vi "Move.vi"(8 "error in (no error)":errorcluster, 11 "AISAS Mech in":refnum<class "AISAS Mech.lvclass">) -> (0 "error out":errorcluster, 3 "AISAS Mech out":refnum<class "AISAS Mech.lvclass">, 5 "status log":string)   [LabVIEW 2014, in "AISAS Mech.lvclass"]
uses:
  AISAS Mech.lvclass
  AISAS Mech.lvclass/AISAS Mech.ctl
  motor/Motor status.ctl
  motor/AISAS motor.lvclass
panel:
  out "M name":string
  in  "Abort":bool
  out "Elapsed Time (s)":dbl
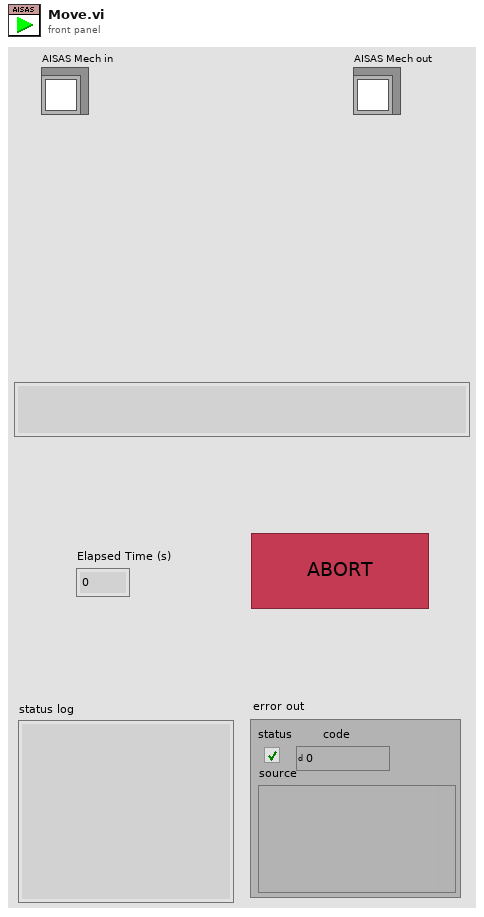
[diagram p1: front panel]
types:
  T1 = typedef "AISAS motor.lvclass/Motor status.ctl" = enum16{"Error", "Ready", "Bussy"}
  T2 = typedef "motor.ctl" = enum32{"Rotation", "Diffuser ", "Focus"}
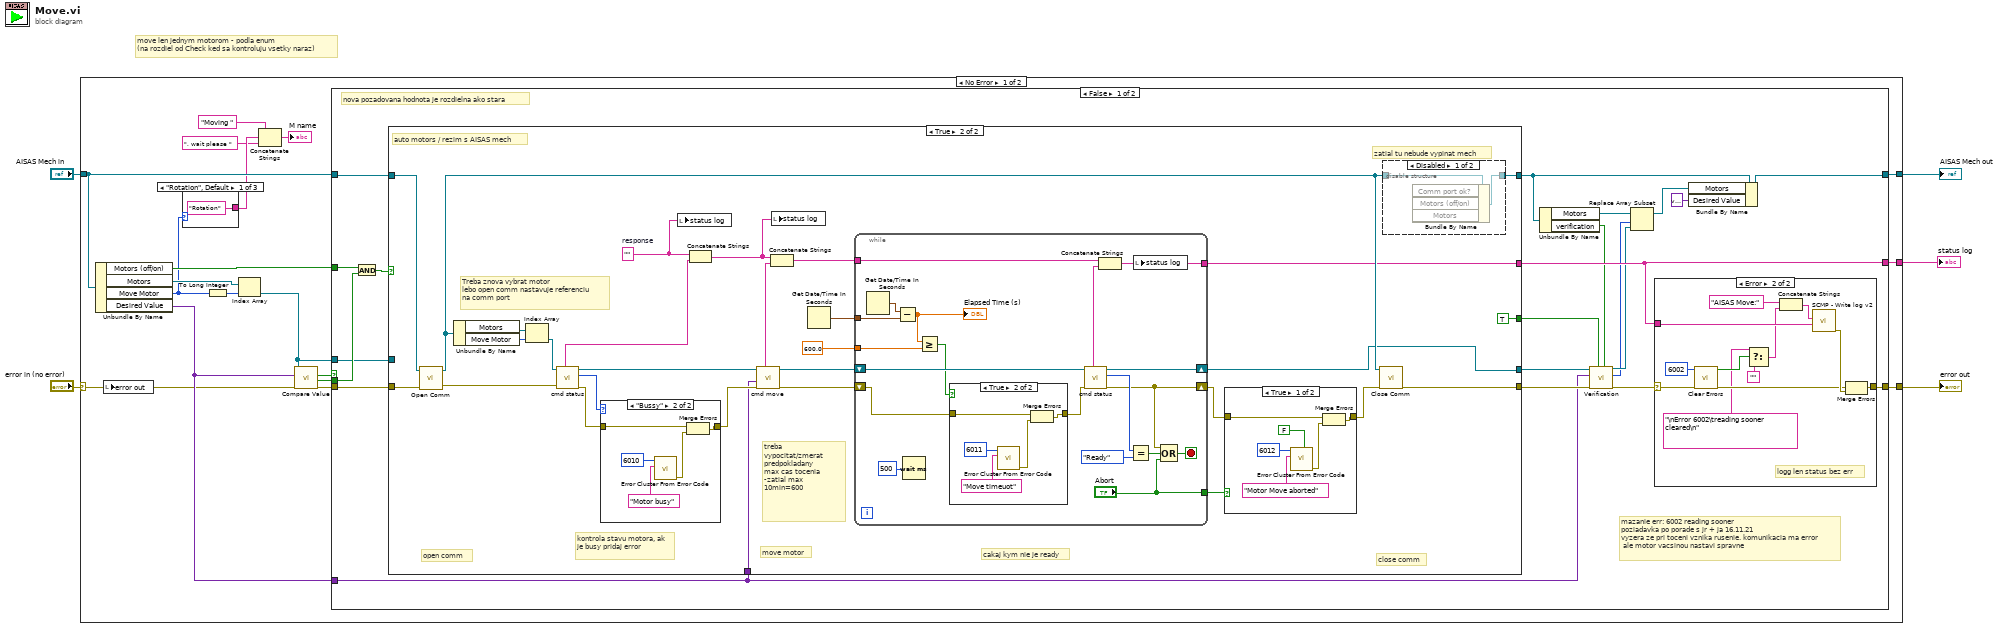
[diagram p0: block diagram]
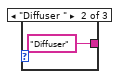
[diagram p2: hidden frame]
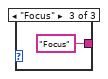
[diagram p3: hidden frame]
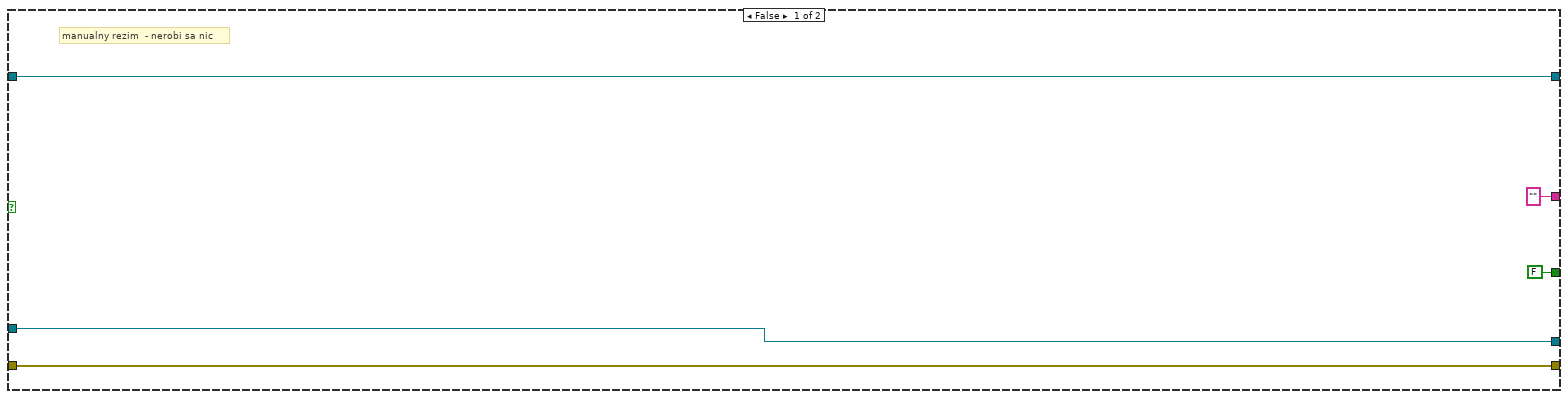
[diagram p5: hidden frame]
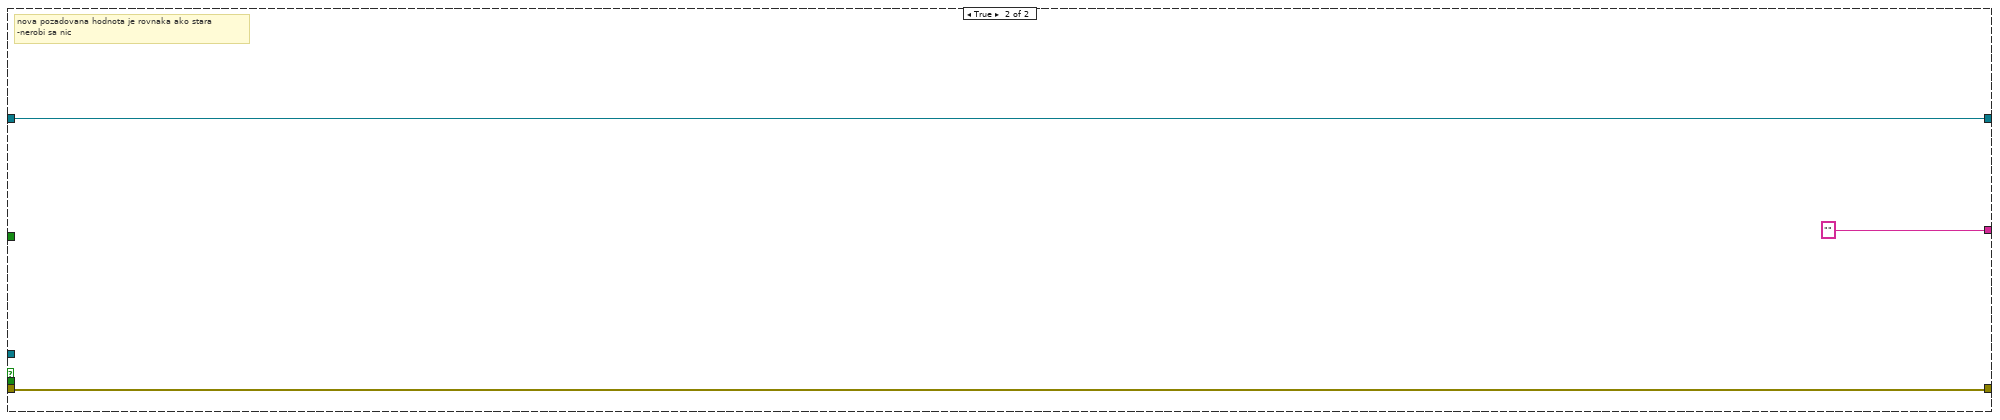
[diagram p10: hidden frame]
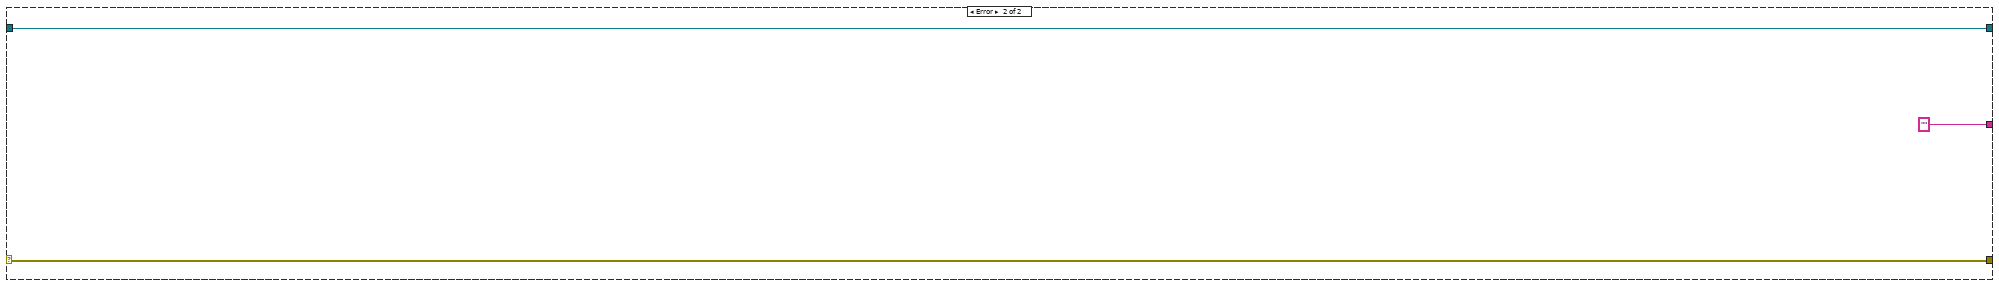
[diagram p11: hidden frame]
diagram:
  # "move len jednym motorom - podla enum \n(na rozdiel od Check ked sa kontroluju vsetky naraz)"
  n1 = case shown="No Error" "error in (no error)" {
    selector: "error in (no error)" -> [w12 w141]
    tunnel: [w23 w141] -> w5
    tunnel: "AISAS Mech in" -> [w21 w140]
    tunnel: [w22 w140] -> w2
    tunnel: [w15 ""] -> w1
    frame No Error {
      n2 = Unbundle By Name(w21) -> ("Motors (off/on)"=w18:bool, "Motors"=w16:refnum<class "AISAS motor.lvclass">[], "Move Motor"=w10:T2, "Desired Value"=w13:variant)
      n3 = local write "error out"(w12) -> ()
      n4 = case shown="\"Rotation\", Default" w10 {
        tunnel: ["Rotation" ("M name") "Diffuser" ("M name") "Focus" ("M name")] -> w8
        frame "Rotation", Default {
        }
        frame "Diffuser " {
        }
        frame "Focus" {
        }
      }
      n5 = To Long Integer(number=w10) -> (32bit integer=w11:i32)
      n6 = Index Array(array=w16, index=w11) -> (element=w14:refnum<class "AISAS motor.lvclass">)
      n7 = Concatenate Strings("Moving " ("M name"), w8, ", wait please " ("M name")) -> (→"M name":string)
      n8 = call "Compare Value.vi"("error in (no error)"=w12, "new Value"=w13, "AISAS motor in"=w14) -> ("error out"=w17:errorcluster, "Motor Ok?"=w19:bool, "same value?"=w20:bool)  [unwired: 3 in, 3 out]
      n9 = case shown="False" w20 {
        tunnel: [w31 w137] -> w23
        tunnel: [w40 w138] -> w22
        tunnel: w21 -> [w47 w138]
        tunnel: w19 -> [w39 _]
        tunnel: w18 -> [w46 _]
        tunnel: w17 -> [w44 w137]
        tunnel: [w30 ""] -> w15
        tunnel: w14 -> [w38 _]
        tunnel: w13 -> [w33 _]
        frame False {
          # "mazanie err: 6002\treading sooner\npoziadavka po porade s jr + ja 16.11.21\nvyzera ze pri toceni vznika rusenie. komunikacia ma error\n ale motor vacsinou nastavi spravne"
          # "nova pozadovana hodnota je rozdielna ako stara"
          n10 = And(x=w46, y=w39) -> (x .and. y?=w45:bool)
          n11 = case shown="True" w45 {
            tunnel: [w64 w74] -> w37
            tunnel: w47 -> [w65 w83]
            tunnel: [w65 w94] -> w41
            tunnel: w44 -> [w64 w85]
            tunnel: [w62 w78] -> w36
            tunnel: ["" w67] -> w30
            tunnel: w38 -> [w62 _]
            tunnel: [FALSE ("Motor (man/auto)") TRUE ("Motor (man/auto)")] -> w35
            tunnel: w33 -> [_ w75]
            frame False {
              # "manualny rezim  - nerobi sa nic"
            }
            frame True {
              w70 = ""  # response
              # "Treba znova vybrat motor\nlebo open comm nastavuje referenciu\nna comm port"
              # "close comm"
              # "cakaj kym nie je ready"
              # "move motor"
              # "kontrola stavu motora, ak je busy pridaj error"
              # "zatial tu nebude vypinat mech"
              # "treba \nvypocitat/zmerat \npredpokladany\nmax cas tocenia\n-zatial max 10min=600"
              # "auto motors / rezim s AISAS mech"
              # "open comm"
              n12 = call "Open Comm.vi"("error in (no error)"=w85, "AISAS Mech in"=w83) -> ("error out"=w84:errorcluster, "AISAS Mech out"=w80:refnum<class "AISAS Mech.lvclass">)  [unwired: 7 in, 1 out]
              n13 = Unbundle By Name(w80) -> ("Motors"=w82:refnum<class "AISAS motor.lvclass">[], "Move Motor"=w76:T2)
              n14 = Index Array(array=w82, index=w76) -> (element=w81:refnum<class "AISAS motor.lvclass">)
              n15 = call "cmd status.vi"("error in (no error)"=w84, "motor in"=w81) -> ("error out"=w86:errorcluster, "Motor status"=w79:T1, "motor out"=w93:refnum<class "AISAS motor.lvclass">, "status log"=w89:string)  [unwired: 5 in, 1 out]
              n16 = case shown="\"Bussy\"" w79 {
                tunnel: w86 -> [w130 w133]
                tunnel: [w130 w131] -> w92
                frame "Error", Default {
                }
                frame "Bussy" {
                  n17 = call <vilib>:"Error Cluster From Error Code.vi"("error message (\"\")"="Motor busy" ("error message (\"\")"), "error code (0)"=6010) -> ("error out"=w132:errorcluster)  [unwired: 7 in]
                  n18 = Merge Errors(w133, w132) -> (w131:errorcluster)
                }
              }
              n19 = local write "status log"(w70) -> ()
              n20 = Concatenate Strings(w70, w89) -> (w69:string)
              n21 = call "cmd move.vi"("error in (no error)"=w92, "new Value"=w75, "motor in"=w93) -> ("error out"=w91:errorcluster, "motor out"=w90:refnum<class "AISAS motor.lvclass">, "Log response"=w88:string)  [unwired: 4 in, 2 out]
              n22 = Concatenate Strings(w69, w88) -> (w68:string)
              n23 = local write "status log"(w69) -> ()
              n24 = Get Date/Time In Seconds() -> (seconds since 1Jan1904=w66:timestamp)
              n25 = while {
                shift-right: [w117] -> w72
                shift-left: w91 -> [w106]
                shift-right: [w120] -> w78
                shift-left: w90 -> [w121]
                tunnel: 600.0 ("Time Target (s)") -> [w109]
                tunnel: ["Abort"] -> w73
                tunnel: w68 -> [w114]
                tunnel: [w112] -> w67
                tunnel: w66 -> [w111]
                stop <- w116 stop-if-true
                n26 = Get Date/Time In Seconds() -> (seconds since 1Jan1904=w110:timestamp)
                n27 = Subtract(x=w110, y=w111) -> (x-y=w108:dbl)
                "Elapsed Time (s)" <- w108
                n28 = Wait (ms)(milliseconds to wait=u32 500) -> ()  [unwired: 1 out]
                n29 = Greater Or Equal?(x=w108, y=w109) -> (x >= y?=w107:bool)
                n30 = case shown="True" w107 {
                  tunnel: [w124 w127] -> w122
                  tunnel: w106 -> [w124 w125]
                  frame False {
                  }
                  frame True {
                    n31 = call <vilib>:"Error Cluster From Error Code.vi"("error message (\"\")"="Move timeuot" ("error message (\"\")"), "error code (0)"=6011) -> ("error out"=w126:errorcluster)  [unwired: 7 in]
                    n32 = Merge Errors(w125, w126) -> (w127:errorcluster)
                  }
                }
                n33 = call "cmd status.vi"("error in (no error)"=w122, "motor in"=w121) -> ("error out"=w117:errorcluster, "Motor status"=w119:T1, "motor out"=w120:refnum<class "AISAS motor.lvclass">, "status log"=w113:string)  [unwired: 5 in, 1 out]
                n34 = Concatenate Strings(w114, w113) -> (w112:string)
                n35 = Equal?(x=w119, y=Motor_status."Ready") -> (x = y?=w115:bool)
                n36 = local write "status log"(w112) -> ()
                n37 = Compound Arithmetic op=OR(w117, w115, "Abort") -> (w116:bool)
              }
              n38 = case shown="True" w73 {
                tunnel: w72 -> [w98 w101]
                tunnel: [w96 w101] -> w71
                frame True {
                  n39 = call <vilib>:"Error Cluster From Error Code.vi"("is warning? (False)"=FALSE, "error message (\"\")"="Motor Move aborted" ("error message (\"\")"), "error code (0)"=6012) -> ("error out"=w97:errorcluster)  [unwired: 6 in]
                  n40 = Merge Errors(w98, w97) -> (w96:errorcluster)
                }
                frame False {
                }
              }
              n41 = call "Close Comm.vi"("error in (no error)"=w71, "AISAS Mech"=w80) -> ("error out"=w74:errorcluster)  [unwired: 9 in]
              n42 = disable-structure shown="Disabled" {
                disable-tunnel: w80 -> [w103 w104]
                disable-tunnel: [w102 w104] -> w94
                frame Disabled {
                  n43 = Bundle By Name(cluster=w103) -> (w102:refnum<class "AISAS Mech.lvclass">)  [unwired: 3 in]
                }
                frame Enabled {
                }
              }
            }
          }
          n44 = Unbundle By Name(w41) -> ("Motors"=w43:refnum<class "AISAS motor.lvclass">[], "verification"=w27:bool)
          n45 = call "Verification.vi"("verification"=w27, "Motor\n(man/auto)"=w35, "error in (no error)"=w37, "Value in"=w33, "AISAS motor in"=w36) -> ("error out"=w32:errorcluster, "Motor"=w28:T2, "AISAS motor out"=w29:refnum<class "AISAS motor.lvclass">)  [unwired: 4 in]
          n46 = Replace Array Subset(array=w43, new element=w29, index=w28) -> (w42:refnum<class "AISAS motor.lvclass">[])
          n47 = case shown="Error" w32 {
            selector: w32 -> [w48 w56]
            tunnel: [w48 w58] -> w31
            tunnel: w30 -> [_ w60]
            frame No Error {
            }
            frame Error {
              # "logg len status bez err"
              n48 = call <vilib>:"Clear Errors.vi"("error in (no error)"=w56, "specific error code to clear (0: all)"=6002) -> ("error out"=w55:errorcluster, "specific error cleared?"=w54:bool)  [unwired: 4 in]
              n49 = Select(t="\nError 6002\treading sooner cleared\n" ("data"), s=w54, f="") -> (s? t:f=w51:string)
              n50 = Concatenate Strings("AISAS Move:" ("data"), w51) -> (w52:string)
              n51 = call "SCMP - Write log v2.vi"("data to end"=w60, "data"=w52) -> ("error out"=w59:errorcluster)  [unwired: 7 in, 2 out]
              n52 = Merge Errors(w55, w59) -> (w58:errorcluster)
            }
          }
          n53 = Bundle By Name(cluster=w41, "Motors"=w42, "Desired Value"=variant) -> (w40:refnum<class "AISAS Mech.lvclass">)
        }
        frame True {
          # "nova pozadovana hodnota je rovnaka ako stara\n-nerobi sa nic"
        }
      }
    }
    frame Error {
    }
  }
  "error out" <- w5
  "AISAS Mech out" <- w2
  "status log" <- w1
